vi "Log Wait Inspect Range State.vi"(6 "STATUS":T1, 8 "error in (no error)":errorcluster, 9 "Trig State":bool, 10 "Module Data":T2={"Status String"="", "STATUS"={"Initialized"=FALSE, "Connected"=FALSE, "Ready"=FALSE, "Inspecting"=FALSE, "Position"=0.0, "Status"=0, "Error"=FALSE, "Code"=0, "MC SM State"=0, "M_Ctrl"=0}, "Timer 1"={"Instance Name"="", "On/Off"=FALSE, "Running"=FALSE}, "Timer 2"={"Instance Name"="", "On/Off"=FALSE, "Running"=FALSE}, "Timer 1 Call State"="", "Timer 2 Call State"="", "LED State 1"=FALSE, "LED State 2"=FALSE, "OK to Connect"=FALSE, "Connecting"=FALSE, "Got FW Ver"=FALSE, "Got Tool Type"=FALSE, "Got Tool Cfg"=FALSE, "Got Fmt Params"=FALSE, "Got FPGA Setup"=FALSE, "Got Cycle Count"=FALSE, "Cancel Inspect"=FALSE, "Trig State"=FALSE, "Encoder Count"=0, "Loop Counter"=0, "Start Sample No."=0, "Host SampleData"=refnum, "Inspection Limits"={"MaxSamples"=50800, "PosToStartScan"=50800, "PosToEndScan"=0, "ScanLength"=50800}, "EventLog.lvclass"=refnum, "Prev. Encdr"=0, "Status Update Cnt"=0, "Update Temperature Cnt"=0, "Cycle Count"=0, "data value reference"=refnum, "Final No. of Blks"=0, "CD Success"=FALSE, "FW Ver Maj/Min"=0.0, "FPGA Setup Reply Notifier"=refnum}, 11 "EventLog in":refnum<class "EventLog.lvclass">) -> (0 "error out":errorcluster, 3 "EventLog out":refnum<class "EventLog.lvclass">)   [LabVIEW 2015, in "Tool Module.lvlib"]
uses:
  Tool Module.lvlib
  Event Logger Library/Event Log/EventLog.lvclass
  Module Data--cluster.ctl
  _STATUS Typedef--cluster.ctl
  Timer State Return Typedef.ctl
  _Sample Data Rtn Cluster--typedef.ctl
  _Inspection Limits cluster--typedef.ctl
  Return FPGA Setup Data (Reply Payload)--cluster.ctl
  Tool Typedefs/_FPGA Setup Params Cluster--typedef.ctl
  Tool Typedefs/_FPGA Timing Constraints Cluster--typedef.ctl
  Tool Typedefs/_FPGA Timing Ctrl Cluster--typedef.ctl
  Tool Typedefs/_FPGA Laser Config Cluster--typedef.ctl
  Tool Typedefs/_FPGA Peak Proc Cfg Cluster--typedef.ctl
  Tool Typedefs/_FPGA SPI Cfg Cluster--typedef.ctl
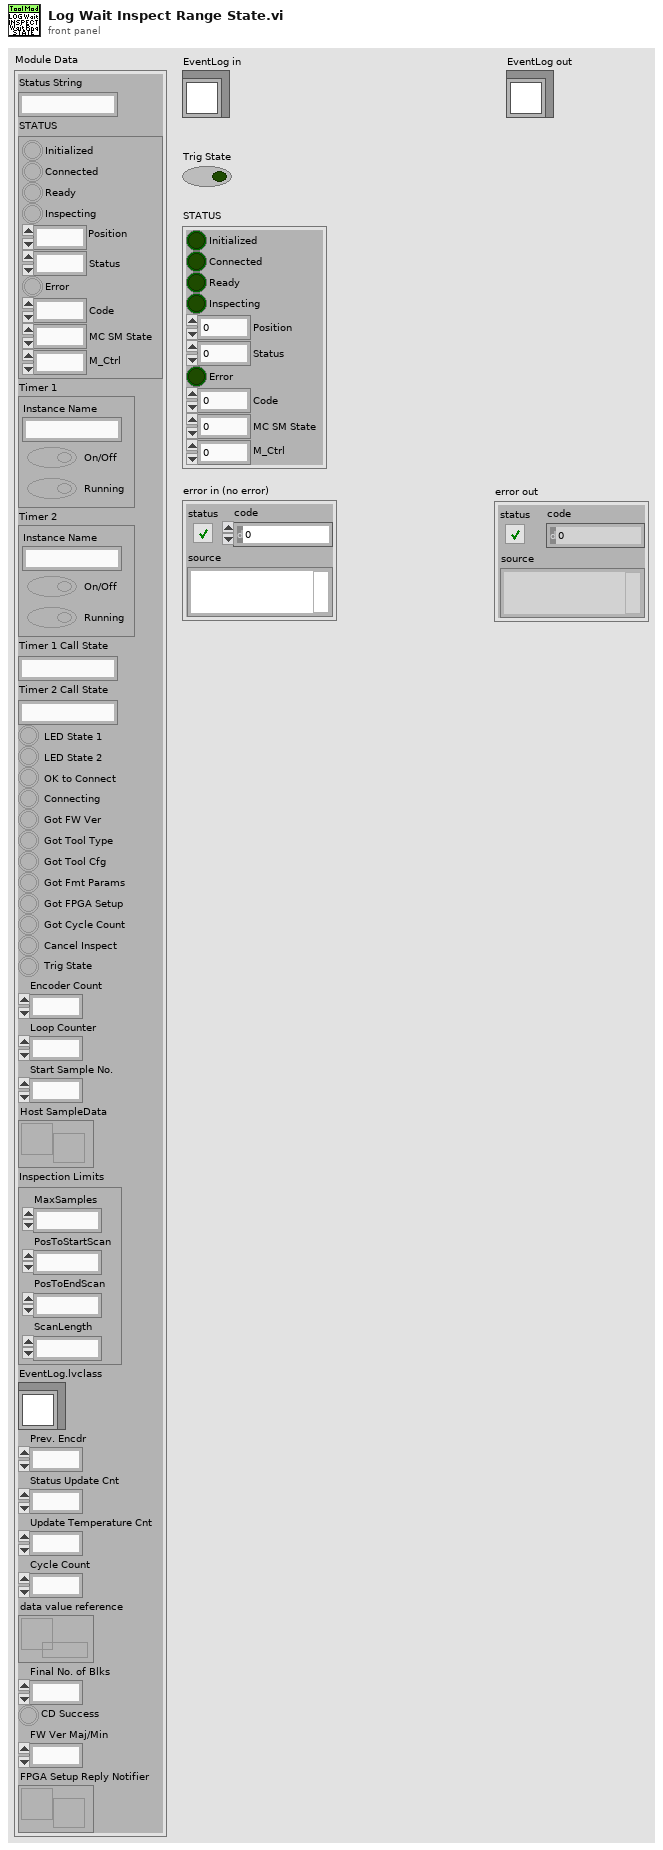
[diagram p1: front panel]
types:
  T1 = typedef "Tool Module.lvlib/_STATUS Typedef--cluster.ctl" = cluster{"Initialized":bool, "Connected":bool, "Ready":bool, "Inspecting":bool, "Position":dbl, "Status":u16, "Error":bool, "Code":i32, "MC SM State":u16, "M_Ctrl":u16}
  T2 = typedef "Tool Module.lvlib/Module Data--cluster.ctl" = cluster{"Status String":string, "STATUS":T1, "Timer 1":T3, "Timer 2":T3, "Timer 1 Call State":string, "Timer 2 Call State":string, "LED State 1":bool, "LED State 2":bool, "OK to Connect":bool, "Connecting":bool, "Got FW Ver":bool, "Got Tool Type":bool, "Got Tool Cfg":bool, "Got Fmt Params":bool, "Got FPGA Setup":bool, "Got Cycle Count":bool, "Cancel Inspect":bool, "Trig State":bool, "Encoder Count":i32, "Loop Counter":i32, "Start Sample No.":u32, "Host SampleData":refnum<notifier>, "Inspection Limits":T4, "EventLog.lvclass":refnum<class "EventLog.lvclass">, "Prev. Encdr":i32, "Status Update Cnt":i32, "Update Temperature Cnt":i32, "Cycle Count":i32, "data value reference":refnum<data-value>, "Final No. of Blks":i32, "CD Success":bool, "FW Ver Maj/Min":dbl, "FPGA Setup Reply Notifier":refnum<notifier>}
  T3 = typedef "Tool Module.lvlib/Timer State Return Typedef.ctl" = cluster{"Instance Name":string, "On/Off":bool, "Running":bool}
  T4 = typedef "Tool Module.lvlib/_Inspection Limits cluster--typedef.ctl" = cluster{"MaxSamples":i32, "PosToStartScan":i32, "PosToEndScan":i32, "ScanLength":i32}
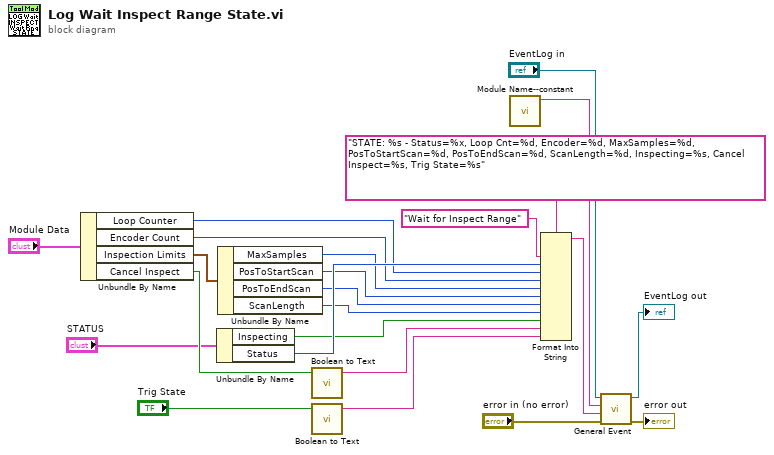
[diagram p0: block diagram]
diagram:
  n1 = Unbundle By Name("Module Data") -> ("Loop Counter"=w5:i32, "Encoder Count"=w4:i32, "Inspection Limits"=w3:T4, "Cancel Inspect"=w2:bool)
  n2 = Unbundle By Name("STATUS") -> ("Inspecting"=w15:bool, "Status"=w23:u16)
  n3 = Unbundle By Name(w3) -> ("MaxSamples"=w17:i32, "PosToStartScan"=w18:i32, "PosToEndScan"=w19:i32, "ScanLength"=w20:i32)
  n4 = call "Boolean to Text.vi"("selector"=w2) -> ("output string"=w21:string)  [unwired: 4 in]
  n5 = call "Boolean to Text.vi"("selector"="Trig State") -> ("output string"=w22:string)  [unwired: 4 in]
  n6 = call "Module Name--constant.vi"() -> ("Module Name"=w8:string)  [unwired: 11 in]
  n7 = Format Into String(format string="STATE: %s - Status=%x, Loop Cnt=%d, Encoder=%d, MaxSamples=%d, PosToStartScan=%d, PosToEndScan=%d, ScanLength=%d, Inspecting=%s, Cancel Inspect=%s, Trig State=%s", "Wait for Inspect Range", w23, w5, w4, w17, w18, w19, w20, w15, w21, w22) -> (resulting string=w14:string)  [unwired: 2 in, 1 out]
  n8 = call "General Event.vi"("error in (no error)"="error in (no error)", "Event Description"=w14, "Event Name"=w8, "EventLog ref"="EventLog in") -> ("error out"=→"error out":errorcluster, "EventLog ref"=→"EventLog out":refnum<class "EventLog.lvclass">)  [unwired: 6 in]
